vi "Join HDC Bank1 DIO.vi"(1 "IN 7:5":fxp<+,3,3> format="%03b", 2 "IN 4":bool, 3 "IN 3:0":fxp<+,4,4> format="%04b") -> (0 "OUT 7:0":u8 format="%08b")   [LabVIEW 2015]
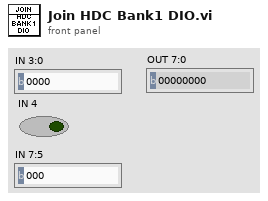
[diagram p1: front panel]
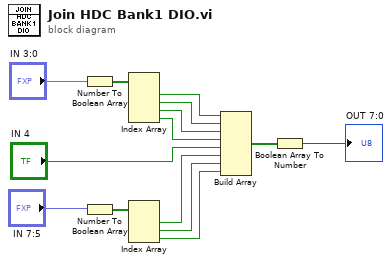
[diagram p0: block diagram]
diagram:
  n1 = Number To Boolean Array(number="IN 3:0") -> (Boolean array=w11:bool[])
  n2 = Number To Boolean Array(number="IN 7:5") -> (Boolean array=w10:bool[])
  n3 = Index Array(array=w11) -> (element #1=w9:bool, element #2=w8:bool, element #3=w7:bool, element #4=w6:bool)  [unwired: 4 in]
  n4 = Index Array(array=w10) -> (element #1=w4:bool, element #2=w3:bool, element #3=w2:bool)  [unwired: 3 in]
  n5 = Build Array(w9, w8, w7, w6, "IN 4", w4, w3, w2) -> (w1:bool[])
  n6 = Boolean Array To Number(Boolean array=w1) -> (number=→"OUT 7:0":u8)
